vi "Agilent DMM Calibrate.vi"(7 "Agilent DMM":T1, 8 "error in (no error)":errorcluster, 10 "Normalization Off? (F)":bool, 11 "VISA Resource Name":refnum<visa-resource-name>) -> (0 "error out":errorcluster {"code" format="%.0x"}, 3 "dup VISA Resource Name":refnum<visa-resource-name>)   [LabVIEW 2011]
uses:
  TypeDefs/Agilent DMM Instrument Info.ctl
  TypeDefs/Agilent DMM Trigger Source.ctl
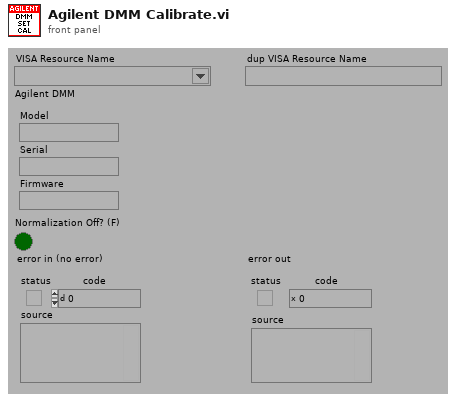
[diagram p1: front panel]
types:
  T1 = typedef "Agilent DMM Instrument Info.ctl" = cluster{"Model":string, "Serial":string, "Firmware":string}
  T2 = typedef "Agilent DMM Trigger Source.ctl" = enum16{"Immediate", "Bus", "External"}
  T3 = typedef "DMM Measurement.ctl" = dbl
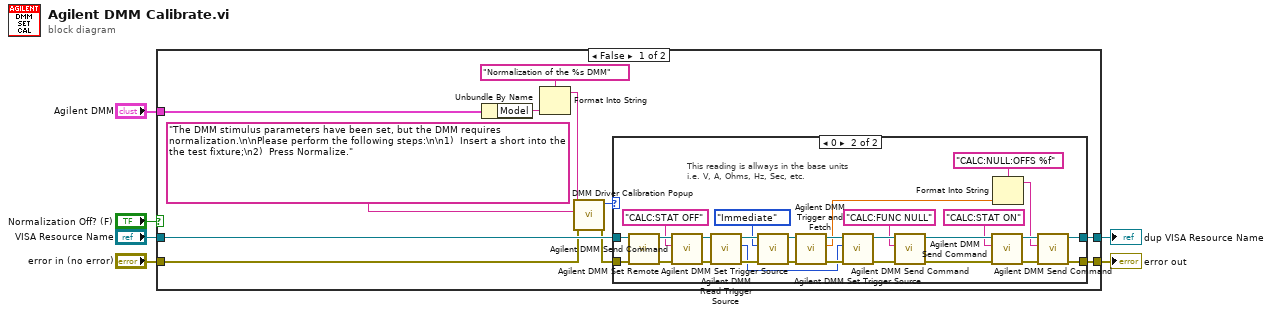
[diagram p0: block diagram]
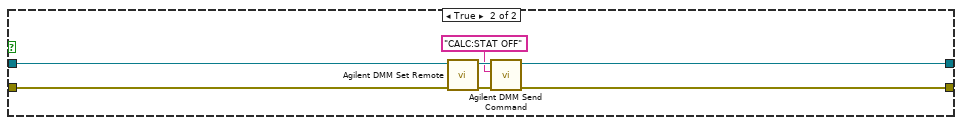
[diagram p3: hidden frame]
diagram:
  n1 = case shown="False" "Normalization Off? (F)" {
    tunnel: "Agilent DMM" -> [w17 _]
    tunnel: "VISA Resource Name" -> [w15 w51]
    tunnel: [w14 w49] -> w4
    tunnel: [w13 w48] -> w3
    tunnel: "error in (no error)" -> [w11 w52]
    frame False {
      n2 = Unbundle By Name(w17) -> ("Model"=w12:string)
      n3 = Format Into String(format string="Normalization of the %s DMM", w12) -> (resulting string=w8:string)  [unwired: 2 in, 1 out]
      n4 = call "DMM Driver Calibration Popup.vi"("error in (no error)"=w11, "Message"="The DMM stimulus parameters have been set, but the DMM requires normalization.\n\nPlease perform the following steps:\n\n1)  Insert a short into the the test fixture;\n2)  Press Normalize.", "Header"=w8) -> ("error out"=w10:errorcluster, "Button"=w9:i32)  [unwired: 7 out]
      n5 = case shown="0" w9 {
        tunnel: w15 -> [w19 w47]
        tunnel: w10 -> [w18 w46]
        tunnel: [w18 w20] -> w14
        tunnel: [w19 w21] -> w13
        frame Default {
        }
        frame 0 {
          # "This reading is allways in the base units\ni.e. V, A, Ohms, Hz, Sec, etc."
          n6 = call "Agilent DMM Set Remote.vi"("error in (no error)"=w46, "VISA Resource Name"=w47) -> ("error out"=w42:errorcluster, "dup VISA Resource Name"=w43:refnum<visa-resource-name>)  [unwired: 8 out]
          n7 = call "Agilent DMM Send Command.vi"("error in (no error)"=w42, "Command"="CALC:STAT OFF" ("T button name (\"OK\")"), "VISA Resource Name"=w43) -> ("error out"=w33:errorcluster, "dup VISA Resource Name"=w32:refnum<visa-resource-name>)  [unwired: 3 in, 4 out]
          n8 = call "Agilent DMM Read Trigger Source.vi"("error in (no error)"=w33, "VISA Resource Name"=w32) -> ("error out"=w40:errorcluster, "Trigger Source"=w34:T2, "dup VISA Resource Name"=w39:refnum<visa-resource-name>)  [unwired: 7 out]
          n9 = call "Agilent DMM Set Trigger Source.vi"("error in (no error)"=w40, "Trigger Source"=Agilent_DMM_Trigger_Source."Immediate", "VISA Resource Name"=w39) -> ("error out"=w37:errorcluster, "dup VISA Resource Name"=w38:refnum<visa-resource-name>)  [unwired: 7 out]
          n10 = call "Agilent DMM Trigger and Fetch.vi"("error in (no error)"=w37, "VISA Resource Name"=w38) -> ("error out"=w35:errorcluster, "Data Reading"=w26:T3, "dup VISA Resource Name"=w36:refnum<visa-resource-name>)  [unwired: 1 in, 6 out]
          n11 = call "Agilent DMM Set Trigger Source.vi"("error in (no error)"=w35, "Trigger Source"=w34, "VISA Resource Name"=w36) -> ("error out"=w28:errorcluster, "dup VISA Resource Name"=w31:refnum<visa-resource-name>)  [unwired: 7 out]
          n12 = call "Agilent DMM Send Command.vi"("error in (no error)"=w28, "Command"="CALC:FUNC NULL" ("T button name (\"OK\")"), "VISA Resource Name"=w31) -> ("error out"=w29:errorcluster, "dup VISA Resource Name"=w30:refnum<visa-resource-name>)  [unwired: 3 in, 4 out]
          n13 = call "Agilent DMM Send Command.vi"("error in (no error)"=w29, "Command"="CALC:STAT ON" ("T button name (\"OK\")"), "VISA Resource Name"=w30) -> ("error out"=w44:errorcluster, "dup VISA Resource Name"=w45:refnum<visa-resource-name>)  [unwired: 3 in, 4 out]
          n14 = Format Into String(format string="CALC:NULL:OFFS %f" ("T button name (\"OK\")"), w26) -> (resulting string=w25:string)  [unwired: 2 in, 1 out]
          n15 = call "Agilent DMM Send Command.vi"("error in (no error)"=w44, "Command"=w25, "VISA Resource Name"=w45) -> ("error out"=w20:errorcluster, "dup VISA Resource Name"=w21:refnum<visa-resource-name>)  [unwired: 3 in, 4 out]
        }
      }
    }
    frame True {
      n16 = call "Agilent DMM Set Remote.vi"("error in (no error)"=w52, "VISA Resource Name"=w51) -> ("error out"=w50:errorcluster, "dup VISA Resource Name"=w54:refnum<visa-resource-name>)  [unwired: 8 out]
      n17 = call "Agilent DMM Send Command.vi"("error in (no error)"=w50, "Command"="CALC:STAT OFF" ("T button name (\"OK\")"), "VISA Resource Name"=w54) -> ("error out"=w49:errorcluster, "dup VISA Resource Name"=w48:refnum<visa-resource-name>)  [unwired: 3 in, 4 out]
    }
  }
  "error out" <- w4
  "dup VISA Resource Name" <- w3
